vi "Read Axis First Frame.vi"(8 "error in":errorcluster, 10 "Acquire Params":T1={"fps"=10, "Compression"=30, "X"=320, "Y"=240, "Enable Color?"=TRUE, "Rotation"=enum."0"}, 11 "address":string="192.168.1.101") -> (0 "error out":errorcluster, 2 "connection ID out":refnum<k5>, 3 "Raw Image Data":string)   [LabVIEW 2017]
panel:
  out "concatenated string":string
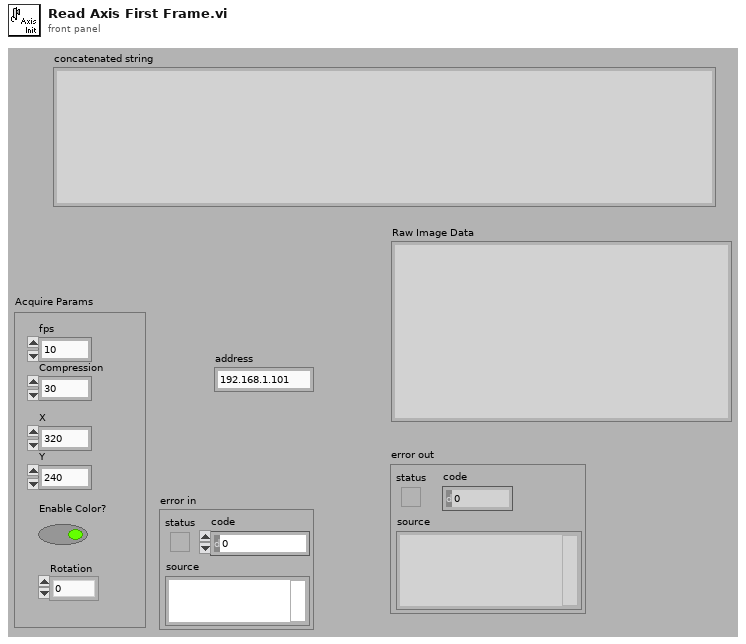
[diagram p1: front panel]
types:
  T1 = cluster{"fps":i32, "Compression":i32, "X":i32, "Y":i32, "Enable Color?":bool, "Rotation":enum16{"0", "90", "180", "270"}}
  T2 = enum16{"Standard", "Buffered", "CRLF", "Immediate"}
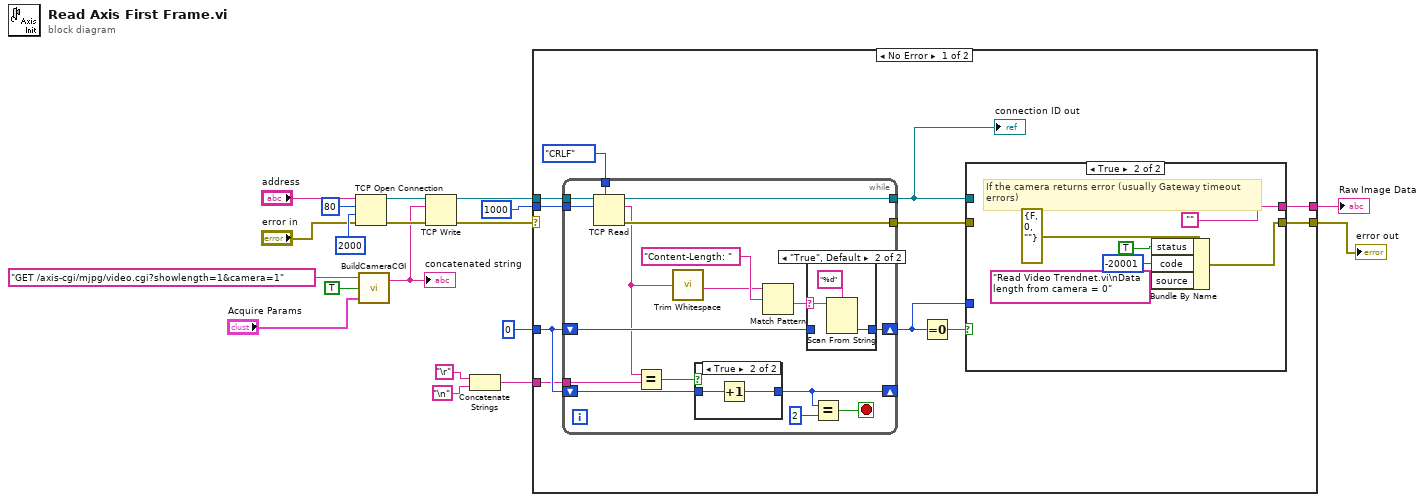
[diagram p0: block diagram]
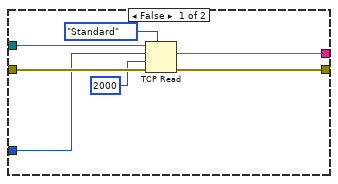
[diagram p4: hidden frame]
diagram:
  n1 = TCP Open Connection(address="address", remote port or service name=u16 80, timeout ms (60000)=2000, error in (no error)="error in") -> (connection ID=w13:refnum<k5>, error out=w11:errorcluster)  [unwired: 1 in]
  n2 = call <vilib>:"BuildCameraCGI.vi"("Acquire Params"="Acquire Params", "FPS?"=TRUE, "Get String"="GET /axis-cgi/mjpg/video.cgi?showlength=1&camera=1") -> ("CGI String"=w10:string)  [unwired: 1 in]
  "concatenated string" <- w10
  n3 = TCP Write(connection ID=w13, data in=w10, error in (no error)=w11) -> (connection ID out=w12:refnum<k5>, error out=w18:errorcluster)  [unwired: 1 in, 1 out]
  n4 = Concatenate Strings("\r", "\n") -> (w2:string)
  n5 = case shown="No Error" w18 {
    selector: w18 -> [_ w68]
    tunnel: [w25 w68] -> w19
    tunnel: w12 -> [w26 _]
    tunnel: 0 -> [w24 _]
    tunnel: 1000 ("bytes to read") -> [w22 _]
    tunnel: w2 -> [w21 _]
    tunnel: [w20 _] -> w1
    frame No Error {
      n6 = while {
        tunnel: w26 -> [w47]
        tunnel: [w46] -> w29
        tunnel: [w45] -> w28
        shift-right: [w41] -> w27
        shift-left: w24 -> [w40]
        shift-right: [w36] -> _
        shift-left: w24 -> [w38]
        tunnel: T2."CRLF" ("mode (standard)") -> [w33]
        tunnel: w22 -> [w32]
        tunnel: w21 -> [w31]
        stop <- w37 stop-if-true
        n7 = TCP Read(connection ID=w47, bytes to read=w32, 7:w33) -> (connection ID out=w46:refnum<k5>, data out=w34:string, error out=w45:errorcluster)  [unwired: 2 in]
        n8 = Equal?(x=w34, y=w31) -> (x = y?=w39:bool)
        n9 = call <vilib>:"Trim Whitespace.vi"("string"=w34) -> ("trimmed string"=w43:string)  [unwired: 1 in]
        n10 = case shown="True" w39 {
          tunnel: w38 -> [w48 w50]
          tunnel: [w48 w49] -> w36
          frame False {
          }
          frame True {
            n11 = Increment(x=w50) -> (x+1=w49:i32)
          }
        }
        n12 = Match Pattern(string=w43, regular expression="Content-Length: ") -> (after substring=w42:string)  [unwired: 1 in, 3 out]
        n13 = case shown="\"True\", Default" w42 {
          selector: w42 -> [_ w52]
          tunnel: [w51 w53] -> w41
          tunnel: w40 -> [w51 _]
          frame "" {
          }
          frame "True", Default {
            n14 = Scan From String(format string="%d", input string=w52) -> (output 1=w53:i32)  [unwired: 3 in, 3 out]
          }
        }
        n15 = Equal?(x=w36, y=2) -> (x = y?=w37:bool)
      }
      "connection ID out" <- w29
      n16 = Equal To 0?(x=w27) -> (x = 0?=w30:bool)
      n17 = case shown="True" w30 {
        tunnel: w29 -> [w61 _]
        tunnel: w28 -> [w60 _]
        tunnel: [w59 w67] -> w25
        tunnel: [w55 ""] -> w20
        tunnel: w27 -> [w56 _]
        frame False {
          n18 = TCP Read(connection ID=w61, bytes to read=w56, error in (no error)=w60, 7:T2."Standard" ("mode (standard)"), 9:2000 ("timeout ms (25000)")) -> (data out=w55:string, error out=w59:errorcluster)  [unwired: 1 out]
        }
        frame True {
          # "If the camera returns error (usually Gateway timeout\nerrors)"
          n19 = Bundle By Name(cluster=errorcluster {"status"=FALSE, "code"=0, "source"=""} ("error in"), "status"=TRUE, "code"=-20001, "source"="Read Video Trendnet.vi\nData length from camera = 0") -> (w67:errorcluster)
        }
      }
    }
    frame Error {
    }
  }
  "error out" <- w19
  "Raw Image Data" <- w1
